vi "GetDataValBwTime.vi"(5 "Time End":dbl, 7 "Time Begin":dbl, 8 "error in (no error)":errorcluster, 10 "Name":string, 11 "ExpData in":refnum<class "ExpData.lvclass">) -> (0 "error out":errorcluster, 1 "Time Inbetween":dbl[](array[numeric]), 2 "Data Inbetween":dbl[][](graph), 3 "ExpData out":refnum<class "ExpData.lvclass">, 4 "ColHeaders":string[](array[string]))   [LabVIEW 2015, in "ExpData.lvclass"]
uses:
  ExpData.lvclass
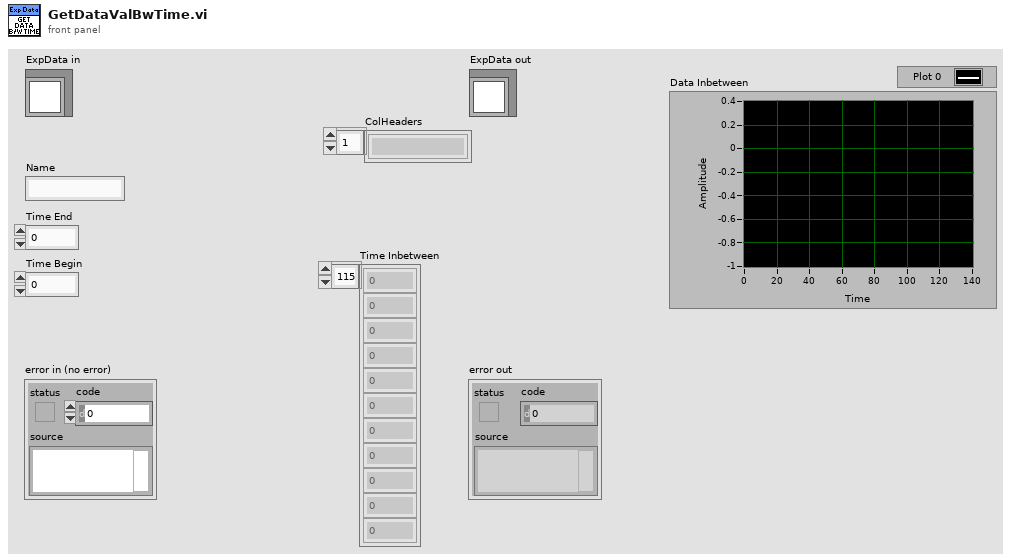
[diagram p1: front panel]
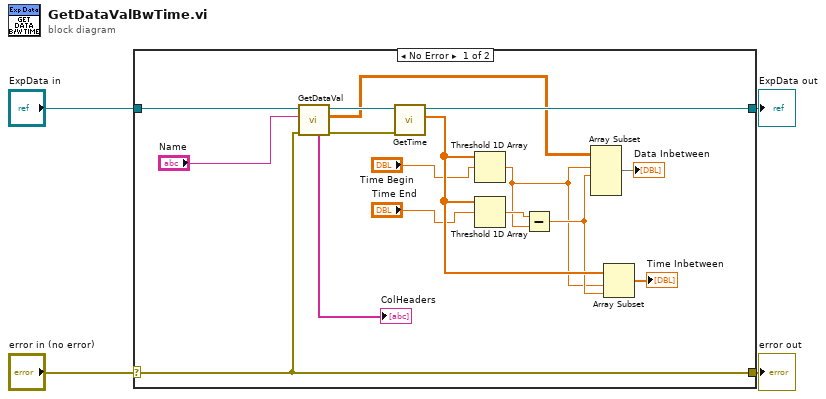
[diagram p0: block diagram]
diagram:
  n1 = case shown="No Error" "error in (no error)" {
    selector: "error in (no error)" -> [w18 w22]
    tunnel: [w18 w22] -> w3
    tunnel: [w16 w21] -> w1
    tunnel: "ExpData in" -> [w20 w21]
    frame No Error {
      n2 = call "GetDataVal.vi"("error in (no error)"=w18, "Name"="Name", "CarexMData in"=w20) -> ("error out"=w14:errorcluster, "Data"=w13:dbl[][], "CarexMData out"=w17:refnum<class "ExpData.lvclass">, "ColHeaders"=→"ColHeaders":string[])  [unwired: 5 in]
      n3 = call "GetTime.vi"("error in (no error)"=w14, "CarexMData in"=w17) -> ("Time"=w10:dbl[], "CarexMData out"=w16:refnum<class "ExpData.lvclass">)  [unwired: 7 in, 1 out]
      n4 = Threshold 1D Array(2:"Time Begin", 3:w10) -> (0:w5:dbl)  [unwired: 1 in]
      n5 = Threshold 1D Array(2:"Time End", 3:w10) -> (0:w12:dbl)  [unwired: 1 in]
      n6 = Subtract(x=w12, y=w5) -> (x-y=w6:dbl)
      n7 = Array Subset(array=w13, index (row)=w5, length (row)=w6) -> (→"Data Inbetween":dbl[][])  [unwired: 2 in]
      n8 = Array Subset(array=w10, index=w5, length=w6) -> (→"Time Inbetween":dbl[])
    }
    frame Error {
    }
  }
  "error out" <- w3
  "ExpData out" <- w1
